vi "SubVI_Encontrar_angulos.vi"(1 "vetor_P":dbl[](array[numeric])) -> (0 "ângulos de Juntas":T1)   [LabVIEW 2017]
panel:
  out "angulos 2":T1
  out "angulos 1":T1
  out "a2":dbl
  out "a1":dbl
  out "a3":dbl
  out "d4":dbl=3.0
  # "ROTINA DE CÔMPUTO\nDE CINEMÁTICA INVERSA\nPELO MÉTODO ALGÉBRICO"
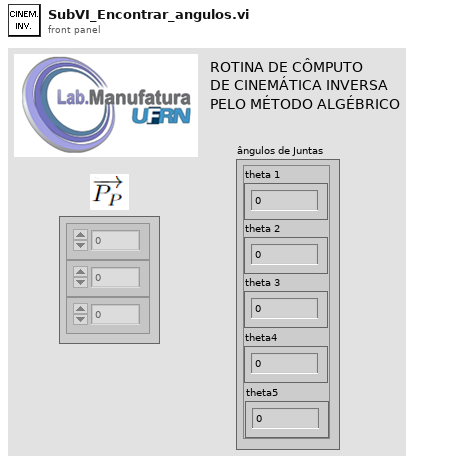
[diagram p1: front panel]
types:
  T1 = cluster{"theta 1":dbl, "theta 2":dbl, "theta 3":dbl, "theta5":dbl, "theta4":dbl}
  T2 = cluster{"Px":dbl, "Py":dbl, "Pz":dbl, "d4":dbl, "a3":dbl, "theta1(rad)":dbl, "a1":dbl, "a2":dbl, "theta1(Graus)":dbl, "theta3.1(Graus)":dbl, "theta3.2(Graus)":dbl, "theta5.1(Graus)":dbl, "theta5.2(Graus) ":dbl, "theta2.1 (Graus)":dbl, "theta2.2 (Graus)":dbl, "theta4 (Graus)":dbl}
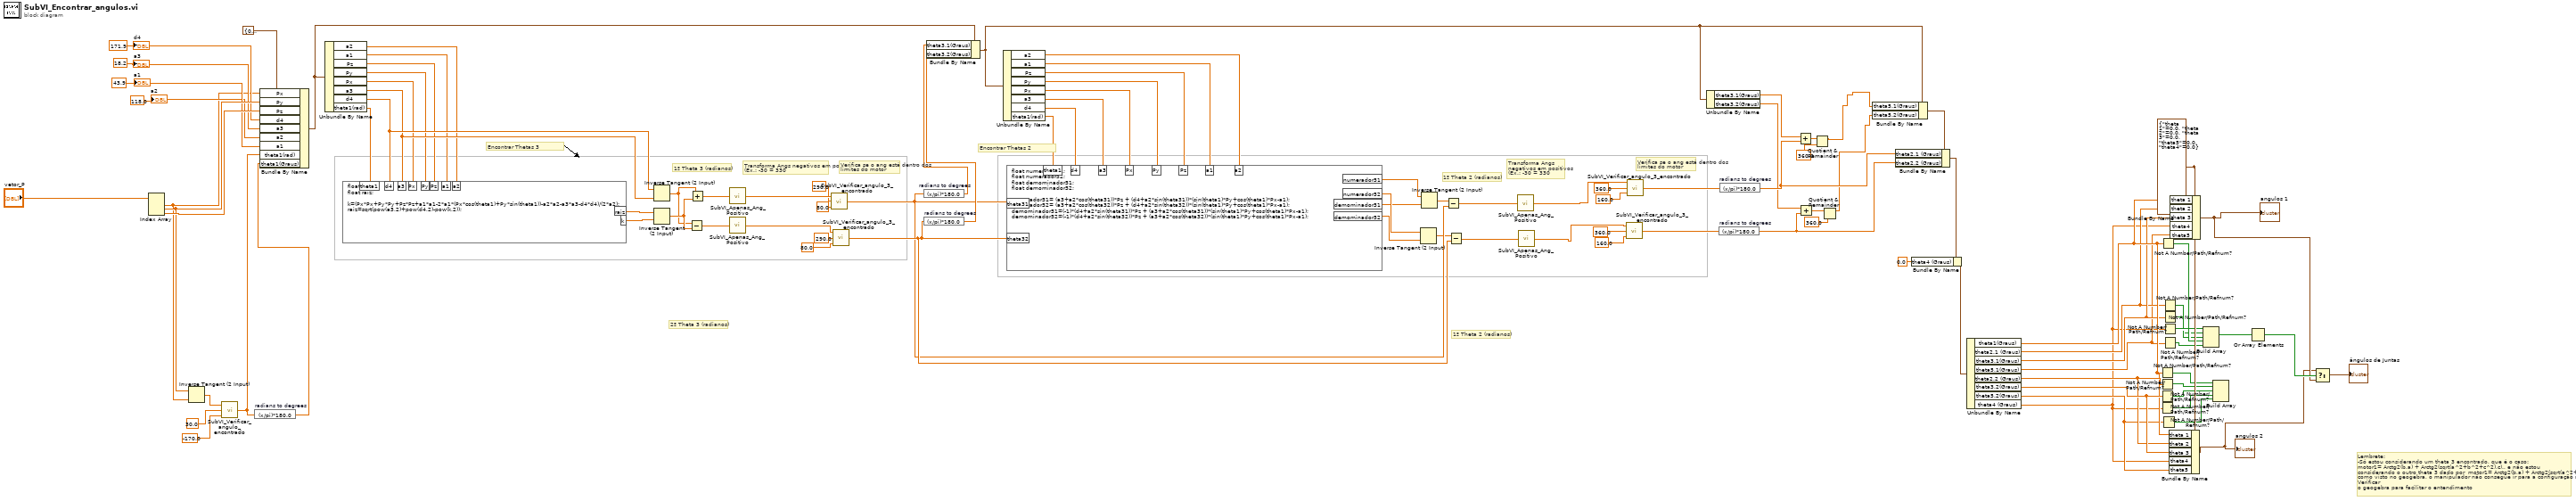
[diagram p0: block diagram]
diagram:
  w100 = T1 {"theta 1"=0.0, "theta 2"=0.0, "theta 3"=0.0, "theta5"=0.0, "theta4"=0.0} ("input cluster")
  w46 = 118.0 ("input variable")
  w47 = 43.9 ("input variable")
  w63 = 18.2 ("input variable")
  w61 = 171.9 ("input variable")
  # "Lembrete:\n-Só estou considerando um theta 3 encontrado, que é o caso:\nmotor1= Arctg2(b,a) + Arctg2(sqrt(a^2+b^2+c^2),c)., e não estou\nconsiderando o outro theta 3 dado por  motor1= Arctg2(b,a) + Arctg2(sqrt(a^2+b^2+c^2),c), pois\ncomo visto no geogebra, o manipulador não consegue ir para a configuração mostrada para m2. Verificar\no geogebra para facilitar o entendimento"
  # "Verifica se o ang está dentro dos limites do motor"
  # "Transforma Angs negativos em positivos\n(Ex.: -30 = 330"
  # "1º Theta 2 (radianos)"
  # "1º Theta 2 (radianos)"
  # "Encontrar Thetas 2"
  # "Verifica se o ang está dentro dos limites do motor"
  # "Transforma Angs negativos em positivos\n(Ex.: -30 = 330"
  # "2º Theta 3 (radianos)"
  # "1º Theta 3 (radianos)"
  # "Encontrar Thetas 3"
  n1 = Index Array(array="vetor_P") -> (element #1=w14:dbl, element #2=w65:dbl, element #3=w66:dbl)  [unwired: 3 in]
  n2 = Inverse Tangent (2 Input)(1:w14, 2:w65) -> (0:w29:dbl)
  n3 = call "SubVI_Verificar_angulo_encontrado.vi"("menor que, dê errado (graus)"=-170.0 ("menor que, dê errado"), "maior que, dê errado (graus)"=30.0 ("maior que, dê errado"), "Angulo encontrado em Rad"=w29) -> ("Resultado(Rad)"=w67:dbl)
  n4 = expression code="(x/pi)*180.0" "radians to degrees"(w67) -> (w82:dbl)
  n5 = Bundle By Name(cluster=T2 {"Px"=0.0, "Py"=0.0, "Pz"=0.0, "d4"=0.0, "a3"=0.0, "theta1(rad)"=0.0, "a1"=0.0, "a2"=0.0, "theta1(Graus)"=0.0, "theta3.1(Graus)"=0.0, "theta3.2(Graus)"=0.0, "theta5.1(Graus)"=0.0, "theta5.2(Graus) "=0.0, "theta2.1 (Graus)"=0.0, "theta2.2 (Graus)"=0.0, "theta4 (Graus)"=0.0} ("input cluster"), "Px"=w14, "Py"=w65, "Pz"=w66, "d4"=w61, "a3"=w63, "a2"=w46, "a1"=w47, "theta1(rad)"=w67, "theta1(Graus)"=w82) -> (w73:T2)
  n6 = Unbundle By Name(w73) -> ("a2"=w52:dbl, "a1"=w51:dbl, "Pz"=w50:dbl, "Py"=w49:dbl, "Px"=w48:dbl, "a3"=w64:dbl, "d4"=w102:dbl, "theta1(rad)"=w62:dbl)
  n7 = formula code="float k;\nfloat raiz;\n\nk=(Px*Px+Py*Py+Pz*Pz+a1*a1-2*a1*(Px*cos(theta1)+Py*sin(theta1))-a2*a2-a3*a3-d4*d4)/(2*a2);\nraiz=sqrt(pow(a3,2)+pow(d4,2)-pow(k,2));"("d4"=w102, "a3"=w64, "Px"=w48, "Py"=w49, "Pz"=w50, "a1"=w51, "a2"=w52, "theta1"=w62) -> ("k"=w16:dbl, "raiz"=w38:dbl)
  n8 = Inverse Tangent (2 Input)(1:w64, 2:w102) -> (0:w17:dbl)
  n9 = Inverse Tangent (2 Input)(1:w16, 2:w38) -> (0:w18:dbl)
  n10 = Subtract(x=w17, y=w18) -> (x-y=w26:dbl)
  n11 = Add(x=w17, y=w18) -> (x+y=w25:dbl)
  n12 = call "SubVI_Apenas_Ang_Positivo.vi"("Ang_entrada"=w26) -> ("Ang_saida"=w37:dbl)
  n13 = call "SubVI_Apenas_Ang_Positivo.vi"("Ang_entrada"=w25) -> ("Ang_saida"=w34:dbl)
  n14 = call "SubVI_Verificar_angulo_3_encontrado.vi"("menor que, dê certo (graus)"=80.0, "maior que, dê certo (graus)"=290.0, "Angulo encontrado em Rad"=w34) -> ("Resultado(Rad)"=w68:dbl)
  n15 = call "SubVI_Verificar_angulo_3_encontrado.vi"("menor que, dê certo (graus)"=80.0, "maior que, dê certo (graus)"=290.0, "Angulo encontrado em Rad"=w37) -> ("Resultado(Rad)"=w70:dbl)
  n16 = expression code="(x/pi)*180.0" "radians to degrees"(w68) -> (w69:dbl)
  n17 = expression code="(x/pi)*180.0" "radians to degrees"(w70) -> (w71:dbl)
  n18 = Bundle By Name(cluster=w73, "theta3.1(Graus)"=w69, "theta3.2(Graus)"=w71) -> (w81:T2)
  n19 = Unbundle By Name(w81) -> ("a2"=w53:dbl, "a1"=w54:dbl, "Pz"=w55:dbl, "Py"=w56:dbl, "Px"=w57:dbl, "a3"=w58:dbl, "d4"=w59:dbl, "theta1(rad)"=w60:dbl)
  n20 = formula code="float numerador31;\nfloat numerador32;\nfloat demominador31;\nfloat demominador32;\n\nnumerador31= (a3+a2*cos(theta31))*Pz + (d4+a2*sin(theta31))*(sin(theta1)*Py+cos(theta1)*Px-a1);\nnumerador32= (a3+a2*cos(theta32))*Pz + (d4+a2*sin(theta32))*(sin(theta1)*Py+cos(theta1)*Px-a1);\ndemominador31=(-1)*(d4+a2*sin(theta31))*Pz + (a3+a2*cos(theta31))*(sin(theta1)*Py+cos(theta1)*Px-a1);\ndemominador32=(-1)*(d4+a2*sin(theta32))*Pz + (a3+a2*cos(theta32))*(sin(theta1)*Py+cos(theta1)*Px-a1);"("d4"=w59, "a3"=w58, "Px"=w57, "Py"=w56, "Pz"=w55, "a1"=w54, "a2"=w53, "theta31"=w68, "theta32"=w70, "theta1"=w60) -> ("numerador31"=w19:dbl, "numerador32"=w21:dbl, "demominador31"=w20:dbl, "demominador32"=w22:dbl)
  n21 = Inverse Tangent (2 Input)(1:w22, 2:w21) -> (0:w24:dbl)
  n22 = Inverse Tangent (2 Input)(1:w20, 2:w19) -> (0:w23:dbl)
  n23 = Subtract(x=w23, y=w68) -> (x-y=w27:dbl)
  n24 = Subtract(x=w24, y=w70) -> (x-y=w28:dbl)
  n25 = call "SubVI_Apenas_Ang_Positivo.vi"("Ang_entrada"=w27) -> ("Ang_saida"=w41:dbl)
  n26 = call "SubVI_Apenas_Ang_Positivo.vi"("Ang_entrada"=w28) -> ("Ang_saida"=w44:dbl)
  n27 = call "SubVI_Verificar_angulo_3_encontrado.vi"("menor que, dê certo (graus)"=160.0, "maior que, dê certo (graus)"=360.0, "Angulo encontrado em Rad"=w44) -> ("Resultado(Rad)"=w75:dbl)
  n28 = call "SubVI_Verificar_angulo_3_encontrado.vi"("menor que, dê certo (graus)"=160.0, "maior que, dê certo (graus)"=360.0, "Angulo encontrado em Rad"=w41) -> ("Resultado(Rad)"=w74:dbl)
  n29 = Unbundle By Name(w81) -> ("theta3.1(Graus)"=w77:dbl, "theta3.2(Graus)"=w78:dbl)
  n30 = expression code="(x/pi)*180.0" "radians to degrees"(w75) -> (w85:dbl)
  n31 = expression code="(x/pi)*180.0" "radians to degrees"(w74) -> (w84:dbl)
  n32 = Add(x=w77, y=w84) -> (x+y=w76:dbl)
  n33 = Add(x=w78, y=w85) -> (x+y=w79:dbl)
  n34 = Quotient & Remainder(x=w76, y=360.0) -> (x-y*floor(x/y)=w2:dbl)  [unwired: 1 out]
  n35 = Quotient & Remainder(x=w79, y=360.0) -> (x-y*floor(x/y)=w1:dbl)  [unwired: 1 out]
  n36 = Bundle By Name(cluster=w81, "theta5.1(Graus)"=w2, "theta5.2(Graus)"=w1) -> (w83:T2)
  n37 = Bundle By Name(cluster=w83, "theta2.1 (Graus)"=w84, "theta2.2 (Graus)"=w85) -> (w12:T2)
  n38 = Bundle By Name(cluster=w12, "theta4 (Graus)"=0.0) -> (w11:T2)
  n39 = Unbundle By Name(w11) -> ("theta1(Graus)"=w97:dbl, "theta2.1 (Graus)"=w95:dbl, "theta3.1(Graus)"=w96:dbl, "theta5.1(Graus)"=w10:dbl, "theta2.2 (Graus)"=w98:dbl, "theta3.2(Graus)"=w99:dbl, "theta5.2(Graus)"=w8:dbl, "theta4 (Graus)"=w6:dbl)
  n40 = Not A Number/Path/Refnum?(number/path/refnum=w97) -> (NaN/Path/Refnum?=w90:bool)
  n41 = Not A Number/Path/Refnum?(number/path/refnum=w98) -> (NaN/Path/Refnum?=w92:bool)
  n42 = Not A Number/Path/Refnum?(number/path/refnum=w99) -> (NaN/Path/Refnum?=w93:bool)
  n43 = Not A Number/Path/Refnum?(number/path/refnum=w6) -> (NaN/Path/Refnum?=w91:bool)
  n44 = Not A Number/Path/Refnum?(number/path/refnum=w97) -> (NaN/Path/Refnum?=w86:bool)
  n45 = Not A Number/Path/Refnum?(number/path/refnum=w8) -> (NaN/Path/Refnum?=w7:bool)
  n46 = Not A Number/Path/Refnum?(number/path/refnum=w95) -> (NaN/Path/Refnum?=w87:bool)
  n47 = Not A Number/Path/Refnum?(number/path/refnum=w96) -> (NaN/Path/Refnum?=w88:bool)
  n48 = Not A Number/Path/Refnum?(number/path/refnum=w6) -> (NaN/Path/Refnum?=w89:bool)
  n49 = Not A Number/Path/Refnum?(number/path/refnum=w10) -> (NaN/Path/Refnum?=w9:bool)
  n50 = Bundle By Name(cluster=w100, "theta 1"=w97, "theta 2"=w98, "theta 3"=w99, "theta4"=w6, "theta5"=w8) -> (w3:T1)
  "angulos 2" <- w3
  n51 = Bundle By Name(cluster=w100, "theta 1"=w97, "theta 2"=w95, "theta 3"=w96, "theta4"=w6, "theta5"=w10) -> (w5:T1)
  "angulos 1" <- w5
  n52 = Build Array(w86, w87, w88, w89, w9) -> (w94:bool[])
  n53 = Build Array(w90, w92, w93, w91, w7) -> ()  [unwired: 1 out]
  n54 = Or Array Elements(Boolean array=w94) -> (logical OR=w101:bool)
  n55 = Select(t=w3, s=w101, f=w5) -> (s? t:f=→"ângulos de Juntas":T1)
  "d4" <- w61
  "a3" <- w63
  "a1" <- w47
  "a2" <- w46
